vi "2_Constant_Output.vi"() -> ()   [LabVIEW 2014]
uses:
  <vilib>/Swabian Instruments/Pulse Streamer/PulseStreamer/typedefs/typedef_OutputState.ctl
  <vilib>/Swabian Instruments/Pulse Streamer/PulseStreamer/typedefs/typedef_ChannelNumber.ctl
  <vilib>/Swabian Instruments/Pulse Streamer/PulseStreamer/PulseStreamer/PulseStreamer.lvclass
  <vilib>/Swabian Instruments/Pulse Streamer/PulseStreamer/PulseStreamer.lvlib
panel:
  in  "ip or hostname":string="pulsestreamer"
  in  "Analog 1":sgl min=-1 max=1
  in  "Analog 0":sgl min=-1 max=1
  in  "Digital 7":bool
  in  "Digital 6":bool
  in  "Digital 5":bool
  in  "Digital 4":bool
  in  "Digital 3":bool
  in  "Digital 2":bool
  in  "Digital 1":bool
  in  "Digital 0":bool
  out "error out":errorcluster
  # "This VI sets the constant values at the Pulse Streamer outputs."
  # "Default host name is 'pulsestreamer' when using DHCP \n(please connect the LAN cable before powering on the device). \nOtherwise the fallback IP is 169.254.8.2 if the device is connected directly to the computer."
  # "Example VI to set a constant output level on all the outputs."
  # "max: +/- 1V"
  # "max: +/- 1V"
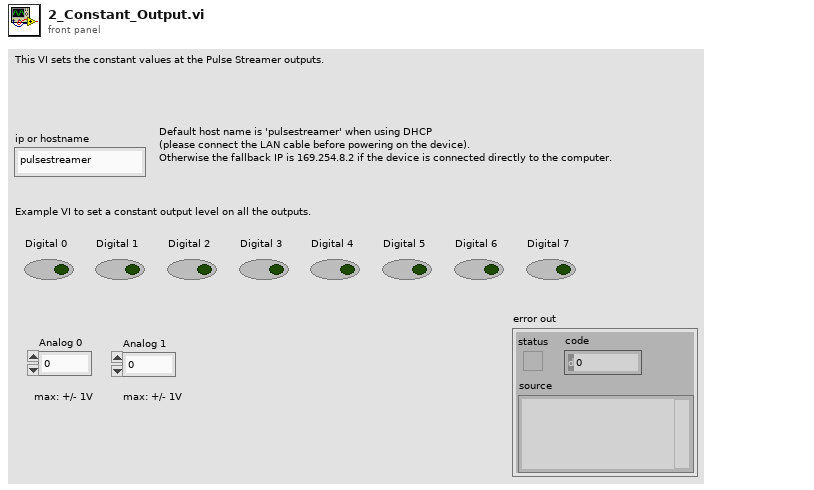
[diagram p1: front panel]
types:
  T1 = typedef "PulseStreamer.lvlib/typedef_OutputState.ctl" = cluster{"channels":T2[], "a0":dbl, "a1":dbl}
  T2 = typedef "PulseStreamer.lvlib/typedef_ChannelNumber.ctl" = i16
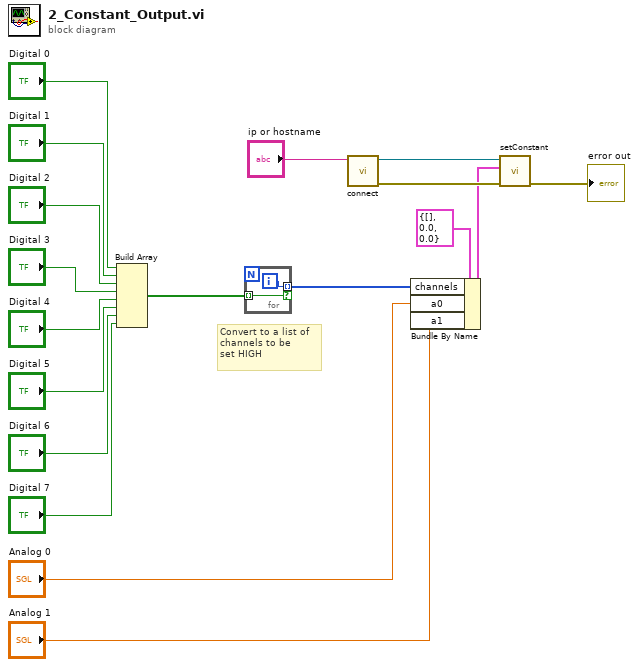
[diagram p0: block diagram]
diagram:
  # "Convert to a list of \nchannels to be \nset HIGH"
  n1 = Build Array("Digital 0", "Digital 1", "Digital 2", "Digital 3", "Digital 4", "Digital 5", "Digital 6", "Digital 7") -> (w6:bool[])
  n2 = for {
    tunnel: [w20] -> w1 mode=indexing if=w19
    tunnel: w6 -> [w19] mode=indexing
    i -> [w20]
  }
  n3 = call <vilib>:"connect.vi"("ip"="ip or hostname") -> ("error out"=w7:errorcluster, "Pulse Streamer out"=w8:refnum<class "PulseStreamer.lvclass">)  [unwired: 9 in]
  n4 = Bundle By Name(cluster=T1 {"channels"=[], "a0"=0.0, "a1"=0.0} ("OutputState"), "channels"=w1, "a0"="Analog 0", "a1"="Analog 1") -> (w4:T1)
  n5 = call-dynamic "setConstant.vi"("error in (no error)"=w7, "outputState"=w4, "Pulse Streamer in"=w8) -> ("error out"=→"error out":errorcluster)  [unwired: 7 in, 1 out]
